vi "dir2tree.vi"(4 "error in":errorcluster, 6 "Dirs":path[](array[path]), 7 "Tree":refnum<vi>) -> (0 "error out":errorcluster, 3 "Tree 2":refnum<vi>)   [LabVIEW 2010]
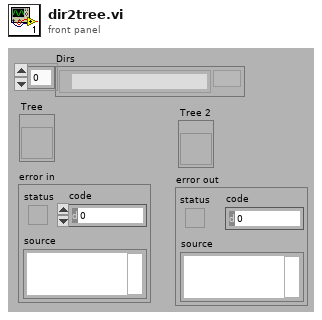
[diagram p1: front panel]
types:
  T1 = cluster{"Left Cell String":string, "Child Text":string[], "Child Tag":string, "Item Indent":i32, "Child Only?":bool, "Glyph Index":i32}
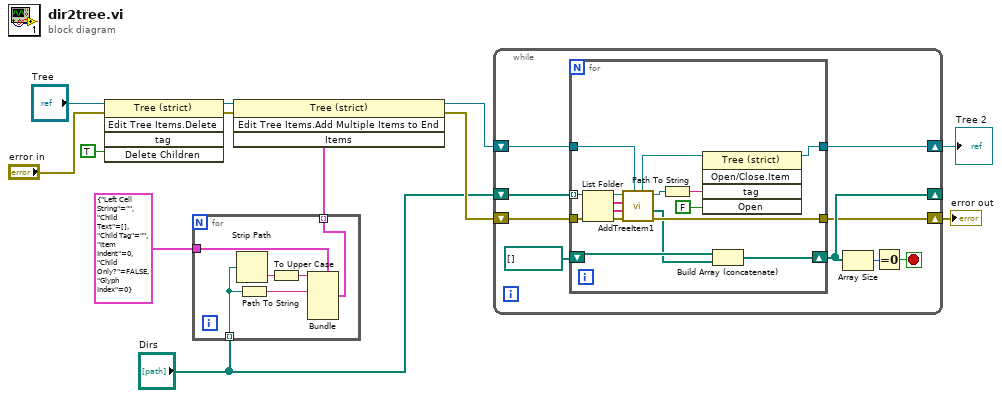
[diagram p0: block diagram]
diagram:
  n1 = invoke class="Tree (strict)" method="Edit Tree Items.Delete"(reference="Tree", error in="error in", "Delete Children"=TRUE ("Delete Children?")) -> (reference out=w2:refnum<vi>, error out=w6:errorcluster)  [unwired: 2 in, 3 out]
  n2 = for {
    tunnel: T1 {"Left Cell String"="", "Child Text"=[], "Child Tag"="", "Item Indent"=0, "Child Only?"=FALSE, "Glyph Index"=0} ("Item") -> [w18]
    tunnel: "Dirs" -> [w17] mode=indexing
    tunnel: [w14] -> w7 mode=indexing
    n3 = Strip Path(path=w17) -> (name=w15:string)  [unwired: 1 out]
    n4 = Path To String(path=w17) -> (string=w16:string)
    n5 = To Upper Case(1:w15) -> (0:w13:string)
    n6 = Bundle(cluster=w18, "Left Cell String"=w13, "Child Tag"=w16) -> (w14:T1)  [unwired: 4 in]
  }
  n7 = invoke class="Tree (strict)" method="Edit Tree Items.Add Multiple Items to End"(reference=w2, error in=w6, "Items"=w7) -> (reference out=w9:refnum<vi>, error out=w5:errorcluster)  [unwired: 1 in, 2 out]
  n8 = while {
    shift-right: [w26] -> _
    shift-left: "Dirs" -> [w23]
    shift-right: [w19] -> w4
    shift-left: w5 -> [w21]
    shift-right: [w20] -> w3
    shift-left: w9 -> [w22]
    stop <- w25 stop-if-true
    n9 = for {
      tunnel: w23 -> [w41] mode=indexing
      shift-right: [w43] -> w26
      shift-left: path[] [] -> [w42]
      tunnel: w22 -> [w37]
      tunnel: [w30] -> w20
      tunnel: w21 -> [w40]
      tunnel: [w38] -> w19
      n10 = List Folder(path=w41, error in=w40) -> (path out=w36:path, filenames=w33:string[], folder names=w34:string[], error out=w39:errorcluster)  [unwired: 2 in]
      n11 = call "AddTreeItem1.vi"("CtlRef 2"=w37, "error in"=w39, "folder names"=w34, "filenames"=w33, "path"=w36) -> ("error out"=w38:errorcluster, "PathArray"=w35:path[], "path out"=w29:path, "CtlRef 3"=w31:refnum<vi>)  [unwired: 1 in]
      n12 = Path To String(path=w29) -> (string=w28:string)
      n13 = invoke class="Tree (strict)" method="Open/Close.Item"(reference=w31, "tag"=w28, "Open"=FALSE ("Open?")) -> (reference out=w30:refnum<vi>)  [unwired: 2 in, 4 out]
      n14 = Build Array (concatenate)(w42, w35) -> (w43:path[])
    }
    n15 = Array Size(array=w26) -> (size(s)=w27:i32)
    n16 = Equal To 0?(x=w27) -> (x = 0?=w25:bool)
  }
  "error out" <- w4
  "Tree 2" <- w3
